vi "DAQ Configuration.vi"(8 "error in":errorcluster) -> (0 "error out":errorcluster, 2 "DUT 2 nReset":refnum<k21>, 3 "DUT 1 nReset":refnum<k21>, 10 "DUT 2 Pinout":refnum<k21>, 11 "DUT 1 Pinout":refnum<k21>)   [LabVIEW 2018]
uses:
  <vilib>/DAQmx/create/channels.llb/DAQmx Create Channel (DI-Digital Input).vi
  <vilib>/DAQmx/create/channels.llb/DAQmx Create Channel (DO-Digital Output).vi
panel:
  # "Configure DAQ Pin\n\nPin Function | DUT Pin Number|     PXI Resource     | DUT 1 | DUT 2 |\nNRESET          |\t             22\t            |  PXIe-6363 (DAQ) |\t  P0.0   |\t \tP0.8  |\nMCU_PA11    |\t             03\t            |  PXIe-6363 (DAQ) |\t  P0.1   |\t \tP0.9  |\nMCU_PB11    |\t             06\t            |  PXIe-6363 (DAQ) |\t  P0.2   |\t P0.10 |\nMCU_PB0      |\t             07             |  PXIe-6363 (DAQ) |\t  P0.3   | \tP0.11 |\nMCU_PA8      |\t             09             |  PXIe-6363 (DAQ) |\t  P0.4   | \tP0.12 |\nMCU_PA5      |\t             10             |  PXIe-6363 (DAQ) |\t  P0.5   | \tP0.13 |\nMCU_PA3      |\t             11             |  PXIe-6363 (DAQ) |\t  P0.6   | \tP0.14 |\nMCU_PA1      |\t             12             |  PXIe-6363 (DAQ) |\t  P0.7   | \tP0.15 |\nMCU_PB10    |\t             13             |  PXIe-6363 (DAQ) |\t  P1.0   | \tP0.16 |\nMCU_PA6      |\t             14             |  PXIe-6363 (DAQ) |\t  P1.1   | \tP0.17 |\nMCU_PA4      |\t             15             |  PXIe-6363 (DAQ) |\t  P1.2   | \tP0.18 |\nMCU_PA2      |\t             17             |  PXIe-6363 (DAQ) |\t  P1.3   | \tP0.19 |\nMCU_PA0      |\t             18             |  PXIe-6363 (DAQ) |\t  P1.4   | \tP0.20 |\nMCU_PB5      |\t             20             |  PXIe-6363 (DAQ) |\t  P1.5   | \tP0.21 |\nMCU_PC15    |\t             25             |  PXIe-6363 (DAQ) |\t  P1.6   | \tP0.22 |\nMCU_PC14    |\t             26             |  PXIe-6363 (DAQ) |\t  P1.7   | \tP0.23 |\nMCU_PB1      |\t             28             |  PXIe-6363 (DAQ) |\t  P2.0   | \tP0.24 |\nMCU_PB7      |\t             29             |  PXIe-6363 (DAQ) |\t  P2.1   | \tP0.25 |\nMCU_PB6      |\t             30             |  PXIe-6363 (DAQ) |\t  P2.2   | \tP0.26 |\nMCU_PA12    |\t             31             |  PXIe-6363 (DAQ) |\t  P2.3   | \tP0.27 |"
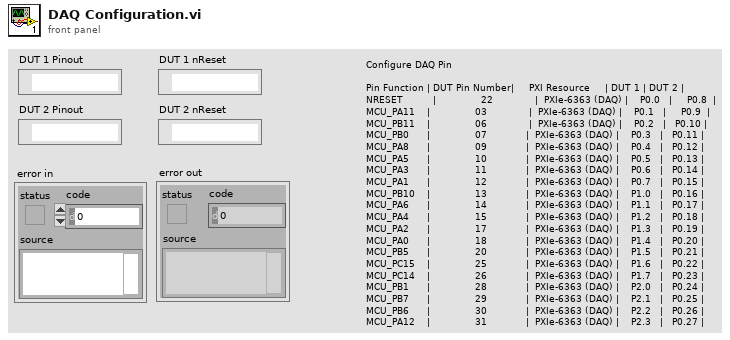
[diagram p1: front panel]
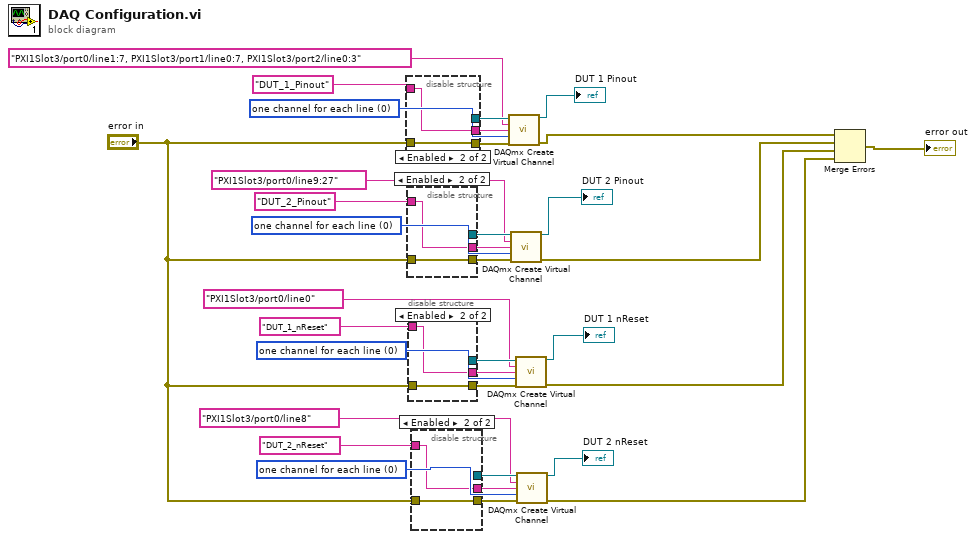
[diagram p0: block diagram]
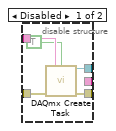
[diagram p2: hidden frame]
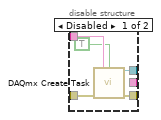
[diagram p3: hidden frame]
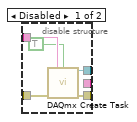
[diagram p4: hidden frame]
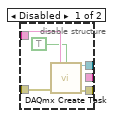
[diagram p5: hidden frame]
diagram:
  w9 = 0 items=["one channel for each line", "one channel for all lines"] ("line grouping")
  w12 = 0 items=["one channel for each line", "one channel for all lines"] ("line grouping")
  w15 = 0 items=["one channel for each line", "one channel for all lines"] ("line grouping")
  w18 = 0 items=["one channel for each line", "one channel for all lines"] ("line grouping")
  n1 = disable-structure shown="Enabled" {
    disable-tunnel: "error in" -> [w39 w40]
    disable-tunnel: [w38 w40] -> w32
    disable-tunnel: [w37 _] -> w27
    disable-tunnel: "DUT_1_Pinout" ("name to assign") -> [w36 w41]
    disable-tunnel: [_ w41] -> w4
    frame Disabled {
      n2 = call <vilib>:"DAQmx Create Task.vi"("new task name"=w36, "auto cleanup"=TRUE, "error in"=w39) -> ("task out"=w37:refnum<k21>, "error out"=w38:errorcluster)  [unwired: 11 in]
    }
    frame Enabled {
    }
  }
  n3 = disable-structure shown="Enabled" {
    disable-tunnel: "error in" -> [w46 w47]
    disable-tunnel: [w45 w47] -> w31
    disable-tunnel: [w44 _] -> w28
    disable-tunnel: "DUT_2_Pinout" ("name to assign") -> [w43 w48]
    disable-tunnel: [_ w48] -> w3
    frame Disabled {
      n4 = call <vilib>:"DAQmx Create Task.vi"("new task name"=w43, "auto cleanup"=TRUE, "error in"=w46) -> ("task out"=w44:refnum<k21>, "error out"=w45:errorcluster)  [unwired: 11 in]
    }
    frame Enabled {
    }
  }
  n5 = disable-structure shown="Enabled" {
    disable-tunnel: "error in" -> [w53 w54]
    disable-tunnel: [w52 w54] -> w30
    disable-tunnel: [w51 _] -> w26
    disable-tunnel: "DUT_1_nReset" ("name to assign") -> [w50 w55]
    disable-tunnel: [_ w55] -> w2
    frame Disabled {
      n6 = call <vilib>:"DAQmx Create Task.vi"("new task name"=w50, "auto cleanup"=TRUE, "error in"=w53) -> ("task out"=w51:refnum<k21>, "error out"=w52:errorcluster)  [unwired: 11 in]
    }
    frame Enabled {
    }
  }
  n7 = disable-structure shown="Enabled" {
    disable-tunnel: "error in" -> [w60 w62]
    disable-tunnel: [w59 w62] -> w29
    disable-tunnel: [w58 _] -> w25
    disable-tunnel: "DUT_2_nReset" ("name to assign") -> [w57 w61]
    disable-tunnel: [_ w61] -> w1
    frame Disabled {
      n8 = call <vilib>:"DAQmx Create Task.vi"("new task name"=w57, "auto cleanup"=TRUE, "error in"=w60) -> ("task out"=w58:refnum<k21>, "error out"=w59:errorcluster)  [unwired: 11 in]
    }
    frame Enabled {
    }
  }
  n9 = call-poly <vilib>:"DAQmx Create Virtual Channel.vi"("task in"=w27, "lines"=tag "PXI1Slot3/port0/line1:7, PXI1Slot3/port1/line0:7, PXI1Slot3/port2/line0:3", "name to assign"=w4, "line grouping"=w18, "error in"=w32) -> ("task out"=→"DUT 1 Pinout":refnum<k21>, "error out"=w8:errorcluster)  [unwired: 9 in]
  n10 = call-poly <vilib>:"DAQmx Create Virtual Channel.vi"("task in"=w28, "lines"=tag "PXI1Slot3/port0/line9:27" ("lines 2"), "name to assign"=w3, "line grouping"=w15, "error in"=w31) -> ("task out"=→"DUT 2 Pinout":refnum<k21>, "error out"=w7:errorcluster)  [unwired: 9 in]
  n11 = call-poly <vilib>:"DAQmx Create Virtual Channel.vi"("task in"=w26, "lines"=tag "PXI1Slot3/port0/line0" ("lines 3"), "name to assign"=w2, "line grouping"=w12, "error in"=w30) -> ("task out"=→"DUT 1 nReset":refnum<k21>, "error out"=w6:errorcluster)  [unwired: 9 in]
  n12 = call-poly <vilib>:"DAQmx Create Virtual Channel.vi"("task in"=w25, "lines"=tag "PXI1Slot3/port0/line8" ("lines 4"), "name to assign"=w1, "line grouping"=w9, "error in"=w29) -> ("task out"=→"DUT 2 nReset":refnum<k21>, "error out"=w5:errorcluster)  [unwired: 9 in]
  n13 = Merge Errors(w8, w7, w6, w5) -> (→"error out":errorcluster)
